vi "Main.vi"() -> ()   [LabVIEW 2019]
doc: "The myRIO Project template acquires acceleration data from the onboard accelerometer and displays the changes of acceleration values in a waveform chart."
uses:
  <vilib>/myRIO/Common/Instrument Driver Framework/myRIO v1.0/Encoder/typedefs/Encoder Signal Mode.ctl
  <vilib>/myRIO/Instrument Drivers/Onboard IO/Encoder/typedefs/Encoder Reference.ctl
  <vilib>/myRIO/Common/Instrument Driver Framework/Utilities/typedefs/myRIO Generic Hardware Reference.ctl
  <vilib>/myRIO/Common/Instrument Driver Framework/Utilities/typedefs/Hardware Version Enum.ctl
  <vilib>/myRIO/Common/Instrument Driver Framework/Utilities/typedefs/myRIO v1.0 Reference.ctl
  <vilib>/myRIO/Common/Instrument Driver Framework/Utilities/typedefs/Generic FPGA Reference.ctl
  <vilib>/myRIO/Common/Instrument Driver Framework/myRIO v1.0/Encoder/typedefs/Encoder Channels Enum.ctl
  <vilib>/myRIO/Common/Instrument Driver Framework/myRIO v1.0/Encoder/typedefs/Encoder Configuration v1.0.ctl
  <vilib>/userDefined/High Color/nirio_resource_hc.ctl
  <vilib>/myRIO/Common/Instrument Driver Framework/Utilities/vis/Is FPGA Ref Available.vi
  <vilib>/myRIO/Common/Instrument Driver Framework/myRIO v1.0/Encoder/vis/myRIO v1.1 Open Encoder.vi
  <vilib>/myRIO/Instrument Drivers/Onboard IO/Encoder/vis/Read.vi
  <vilib>/myRIO/Common/Instrument Driver Framework/Utilities/vis/Validate Channels.vi
  <vilib>/myRIO/Common/Instrument Driver Framework/myRIO v1.0/Encoder/vis/myRIO v1.0 Reserve Encoder.vi
  <vilib>/myRIO/Common/Instrument Driver Framework/myRIO v1.0/UART/vis/myRIO v1.0 Close UART.vi
  <vilib>/myRIO/Common/Instrument Driver Framework/myRIO v1.0/Encoder/vis/myRIO v1.0 Build MUX Configuration Encoder.vi
  <vilib>/myRIO/Common/Instrument Driver Framework/myRIO v1.0/Resource Manager/vis/myRIO v1.0 Reserve Channel List.vi
  <vilib>/myRIO/Common/Instrument Driver Framework/myRIO v1.0/Resource Manager/vis/myRIO v1.0 Create Configuration List.vi
  <vilib>/myRIO/Common/Instrument Driver Framework/myRIO v1.0/Resource Manager/vis/myRIO v1.0 Reserve Channel.vi
  <vilib>/myRIO/Common/Instrument Driver Framework/myRIO v1.0/Resource Manager/vis/myRIO v1.0 Unreserve Channel.vi
  <vilib>/myRIO/Common/Instrument Driver Framework/myRIO v1.0/Resource Manager/vis/myRIO v1.0 Build Mutex Name.vi
  <vilib>/Utility/VariantDataType/GetNumericInfo.vi
  <vilib>/Utility/error.llb/Error Cluster From Error Code.vi
  <vilib>/myRIO/Common/Instrument Driver Framework/myRIO v1.0/myRIO v1.1 Open.vi
  <vilib>/myRIO/Common/Instrument Driver Framework/Utilities/vis/IO Manager.vi
  <vilib>/myRIO/Common/Instrument Driver Framework/Utilities/vis/Configuration Manager.vi
  <vilib>/myRIO/Common/Instrument Driver Framework/myRIO v1.0/Resource Manager/vis/myRIO v1.0 Configure IO.vi
  <vilib>/myRIO/Common/Instrument Driver Framework/myRIO v1.0/myRIO v1.0 Close.vi
  <vilib>/myRIO/Common/Instrument Driver Framework/myRIO v1.0/Encoder/vis/myRIO v1.0 Configure Encoder.vi
  <vilib>/myRIO/Common/Instrument Driver Framework/myRIO v1.0/Encoder/vis/myRIO v1.0 Read Encoder.vi
  <vilib>/Utility/file.llb/Write Delimited Spreadsheet (DBL).vi
  <vilib>/myRIO/Common/Instrument Driver Framework/Utilities/vis/FPGA Ref Manager.vi
  <vilib>/myRIO/Common/Instrument Driver Framework/myRIO v1.0/myRIO v1.0 Reset FPGA.vi
  <vilib>/myRIO/Common/Instrument Driver Framework/myRIO v1.0/IRQ/vis/myRIO v1.0 IRQ Info FGV.vi
  <vilib>/myRIO/Common/Instrument Driver Framework/myRIO v1.0/IRQ/vis/myRIO v1.0 Timer IRQ Info FGV.vi
  <vilib>/myRIO/Common/Instrument Driver Framework/myRIO v1.0/IRQ/vis/myRIO v1.0 ISR Agent.vi
  <vilib>/myRIO/Instrument Drivers/Utilities/vis/Reset Index.vi
  <vilib>/myRIO/Common/Instrument Driver Framework/myRIO v1.0/Resource Manager/vis/myRIO v1.0 Block Write Resource Manager.vi
  <vilib>/myRIO/Express VI/Onboard IO/Encoder/Encoder Express VI.xnode
  <vilib>/myRIO/Common/Instrument Driver Framework/myRIO v1.0/Encoder/typedefs/Encoder Count Direction Enum.ctl
  <vilib>/myRIO/Instrument Drivers/Onboard IO/Encoder/vis/myRIO Encoder Open.xnode
  <vilib>/myRIO/Instrument Drivers/Onboard IO/Encoder/Encoder.lvlib
  <vilib>/myRIO/Instrument Drivers/Utilities/Utilities.lvlib
panel:
  in  "-K":dbl=-0.5 format="%#_13g"
  out "pos2":dbl
  out "pos 1":dbl
  in  "p":dbl
  in  "theta":dbl
  out "ref pos 2":dbl
  out "error out":errorcluster
  in  "Stop 2":bool
  out "Direction 1":enum16{"Counting Up", "Counting Down"}(ring)
  out "Overflow? 1":bool
  in  "Reset":bool
  out "Graph 3":cluster{"ref 1":dbl, "rads":dbl}(graph)
  in  "Freq[Hz]":dbl=1000.0
  out "Direction 2":enum16{"Counting Up", "Counting Down"}(ring)
  out "Overflow? 2":bool
  in  "Reset 2":bool
  out "ref pos 1":dbl
  out "Duty Cycle out 2":dbl=0.5
  out "Duty Cycle out":dbl=0.5
  out "Graph 2":cluster{dbl, "x2hat":dbl}(graph)
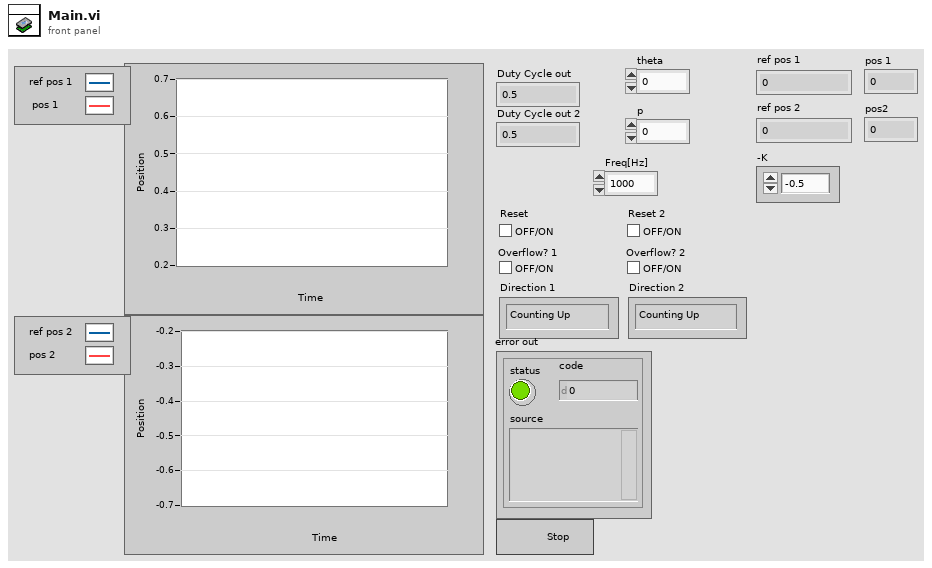
[diagram p1: front panel]
types:
  T1 = typedef "Encoder.lvlib/Encoder Reference.ctl" = cluster{"myRIO Reference":T2, "Encoder Channels Enum":T6}
  T2 = typedef "myRIO Generic Hardware Reference.ctl" = cluster{"myRIO Model":T3, "myRIO Hardware Reference":T4}
  T3 = typedef "Hardware Version Enum.ctl" = enum16{"Unknown", "myRIO-1900", "myRIO-1950", "roboRIO", "NI ELVIS RIO CM", "ELVIS III"}
  T4 = typedef "myRIO v1.0 Reference.ctl" = cluster{"Generic FPGA Reference":T5, "Allow multiple opens":bool}
  T5 = typedef "Generic FPGA Reference.ctl" = refnum<k20>
  T6 = typedef "Encoder Channels Enum.ctl" = enum16{"Not Connected", "C/ENC0", "C/ENC1", "A/ENC", "A/ENC0", "A/ENC1", "A/ENC2", "A/ENC3", "A/ENC4", "A/ENC5", "A/ENC6", "A/ENC7", "A/ENC8", "A/ENC9", "B/ENC", "B/ENC0", "B/ENC1", "B/ENC2", "B/ENC3", "B/ENC4", "B/ENC5", "B/ENC6", "B/ENC7", "B/ENC8", "B/ENC9", "DIO/ENC0", "DIO/ENC1", "DIO/ENC2", "DIO/ENC3", "DIO/ENC4"}
  T7 = typedef "Encoder Signal Mode.ctl" = enum16{"Quadrature phase signal", "Step and direction signal"}
  T8 = typedef "nirio_resource_hc.ctl" = tag
  T9 = typedef "Encoder Count Direction Enum.ctl" = enum16{"Counting Up", "Counting Down"}
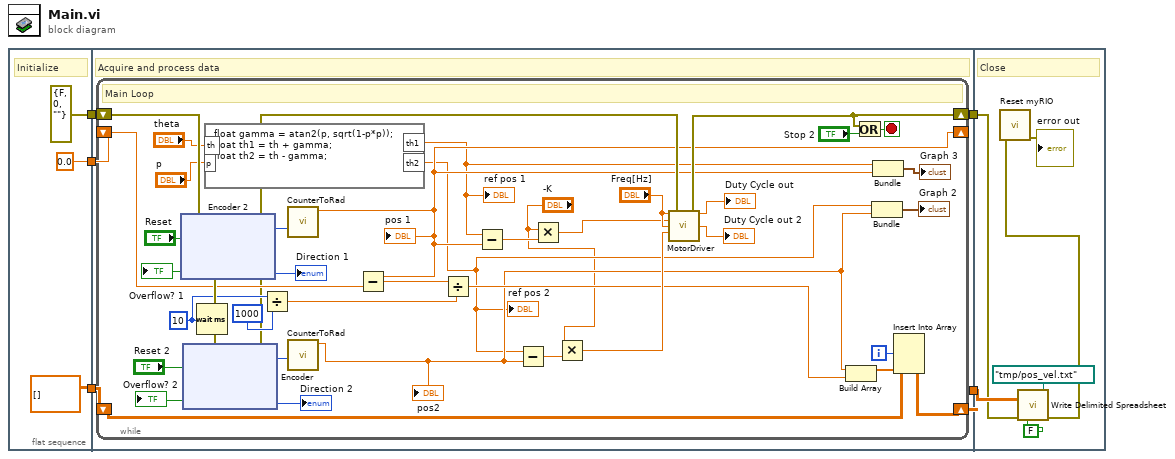
[diagram p0: block diagram]
diagram:
  n1 = flat-sequence {
    tunnel: [errorcluster {"status"=FALSE, "code"=0, "source"=""} ("error in (no error)")] -> w5
    tunnel: [dbl[][] [] ("array")] -> w4
    tunnel: [0.0 ("rads")] -> w3
    tunnel: w5 -> [w13]
    tunnel: w4 -> [w12]
    tunnel: [w11] -> w2
    tunnel: [w10] -> w1
    tunnel: w3 -> [w9]
    tunnel: w2 -> [w149]
    tunnel: w1 -> [w150]
    frame #0 {
      # "Initialize"
    }
    frame #1 {
      # "Acquire and process data"
      n2 = while {
        shift-right: [w24] -> w11
        shift-left: w13 -> [w45]
        shift-right: [w48] -> w10
        shift-left: w12 -> [w47]
        shift-right: [w19] -> _
        shift-left: w9 -> [w35]
        i -> [w44]
        stop <- w52 stop-if-true
        w36 = u32 10 ("milliseconds to wait")
        # "Main Loop"
        n3 = xnode "Encoder 2"("error in (no error)"=w45, "Reset Counter"="Reset") -> ("error out"=w40:errorcluster, "Counter Value"=w34:i32, "Counter Direction"=→"Direction 1":T9, "Overflow?"=→"Overflow? 1":bool)
        n4 = xnode "Encoder"("error in (no error)"=w40, "Reset Counter"="Reset 2") -> ("error out"=w25:errorcluster, "Counter Value"=w33:i32, "Counter Direction"=→"Direction 2":T9, "Overflow?"=→"Overflow? 2":bool)
        n5 = Wait (ms)(milliseconds to wait=w36) -> ()  [unwired: 1 out]
        n6 = formula code="float gamma = atan2(p, sqrt(1-p*p));\nfloat th1 = th + gamma;\nfloat th2 = th - gamma;"("p"="p", "th"="theta") -> ("th1"=w16:dbl, "th2"=w15:dbl)
        "ref pos 1" <- w16
        "ref pos 2" <- w15
        n7 = Divide(x=w36, y=u32 1000) -> (x/y=w39:dbl)
        n8 = call "CounterToRad.vi"("Counter Value"=w34) -> ("rads"=w19:dbl)  [unwired: 10 in]
        "pos 1" <- w19
        n9 = call "CounterToRad.vi"("Counter Value"=w33) -> ("rads"=w22:dbl)  [unwired: 10 in]
        "pos2" <- w22
        n10 = Subtract(x=w19, y=w35) -> (x-y=w38:dbl)
        n11 = Divide(x=w38, y=w39) -> (x/y=w23:dbl)
        n12 = Subtract(x=w16, y=w19) -> (x-y=w29:dbl)
        n13 = Subtract(x=w15, y=w22) -> (x-y=w27:dbl)
        n14 = Multiply(x="-K", y=w29) -> (x*y=w28:dbl)
        n15 = Multiply(x="-K", y=w27) -> (x*y=w26:dbl)
        n16 = call "MotorDriver.vi"("Frequency [Hz]"="Freq[Hz]", "Duty Cycle in"=w28, "Frequency [Hz] 2"="Freq[Hz]", "Duty Cycle in 2"=w26, "error in (no error)"=w25) -> ("Duty Cycle out"=→"Duty Cycle out":dbl, "Duty Cycle out 2"=→"Duty Cycle out 2":dbl, "error out"=w24:errorcluster)  [unwired: 8 in]
        n17 = Build Array(w22, w23) -> (w46:dbl[])
        n18 = Or(x=w24, y="Stop 2") -> (x .or. y?=w52:bool)
        n19 = Bundle(w15, "rads"=w22) -> (→"Graph 2":cluster{dbl, "rads":dbl})  [unwired: 1 in]
        n20 = Bundle(w16, "rads"=w19) -> (→"Graph 3":cluster{dbl, "rads":dbl})  [unwired: 1 in]
        n21 = Insert Into Array(array=w47, index (row)=w44, new element=w46) -> (w48:dbl[][])  [unwired: 1 in]
      }
    }
    frame #2 {
      # "Close"
      n22 = call-poly <vilib>:"Write Delimited Spreadsheet.vi"("file path (dialog if empty)"=path "/tmp/pos_vel.txt", "2D data"=w150, "error in (no error)"=w149, "transpose? (no:F)"=FALSE) -> ("error out"=w148:errorcluster)  [unwired: 10 in, 1 out]
      n23 = call <vilib>:"Reset myRIO.vi"("error in (no error)"=w148) -> ("error out"=→"error out":errorcluster)  [unwired: 10 in]
    }
  }
